vi "ExpLogSaveLoad.vi"   [LabVIEW 2017]
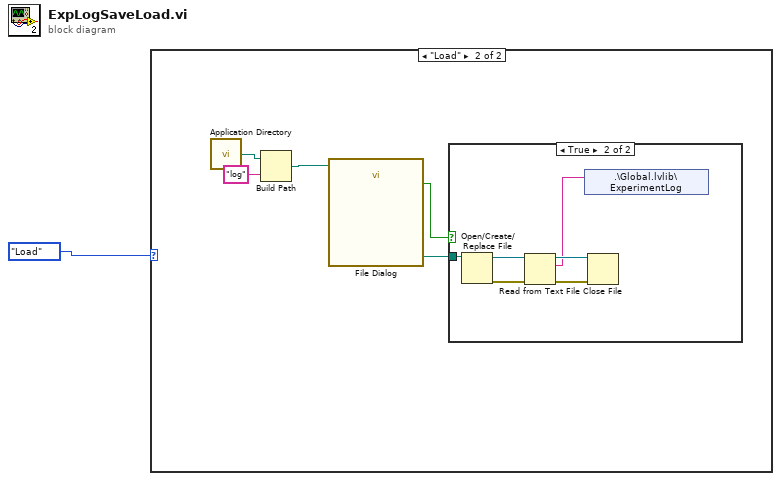
[diagram p0: block diagram]
diagram:
  n1 = case shown="\"Load\"" enum16{"Save", "Load"}."Load" {
    frame "Save", Default {
    }
    frame "Load" {
      n2 = call <vilib>:"Application Directory.vi"() -> ("Application Directory"=w6:path)
      n3 = Build Path(base path=w6, name or relative path="log") -> (appended path=w4:path)
      n4 = call "File Dialog"("start path"=w4) -> ("selected path"=w3:path, "exists"=w2:bool)  [unwired: 11 in, 2 out]
      n5 = case shown="True" w2 {
        tunnel: w3 -> [_ w12]
        frame False {
        }
        frame True {
          n6 = Open/Create/Replace File(file path (use dialog)=w12) -> (refnum out=w11:refnum<file>, error out=w10:errorcluster)  [unwired: 5 in, 1 out]
          n7 = Read from Text File(file (use dialog)=w11, error in=w10) -> (refnum out=w9:refnum<file>, text=w7:string, error out=w8:errorcluster)  [unwired: 2 in, 1 out]
          n8 = shared-variable ".\\Global.lvlib\\ExperimentLog"(w7) -> ()  [unwired: 1 in, 1 out]
          n9 = Close File(refnum=w9, error in=w8) -> ()  [unwired: 2 out]
        }
      }
    }
  }
